vi "Flush Data to Log File.vi"(8 "error in (no error)":errorcluster, 10 "Data Queue":refnum<queue>, 11 "Logging Configuration":T1) -> (0 "error out":errorcluster)   [LabVIEW 2017, in "Logging.lvlib"]
doc: "Flush the data queue of any pending data and write it to the log file. Close the TDMS file reference."
uses:
  Logging.lvlib
  Logging Configuration.ctl
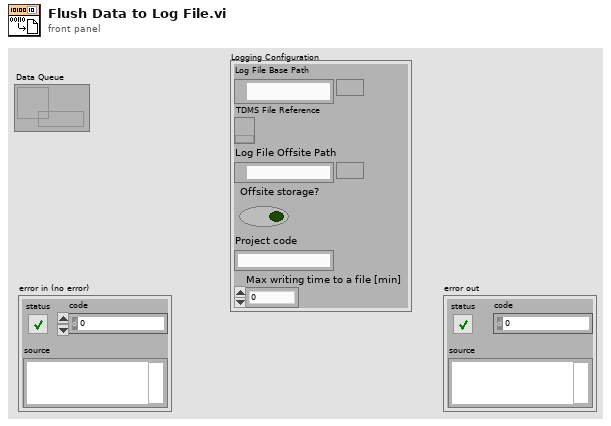
[diagram p1: front panel]
types:
  T1 = typedef "Logging.lvlib/Logging Configuration.ctl" = cluster{"Log File Base Path":path, "TDMS File Reference":refnum<k34>, "Log File Offsite Path":path, "Offsite storage?":bool, "Project code":string, "Max writing time to a file [min]":dbl}
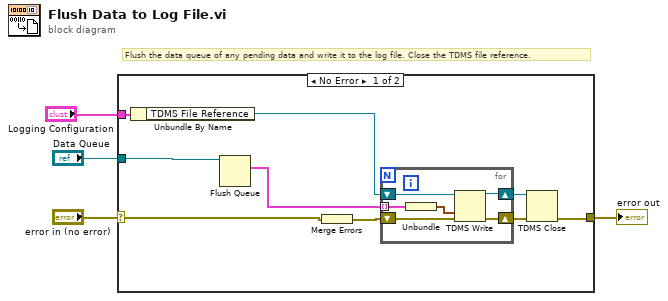
[diagram p0: block diagram]
diagram:
  # "Flush the data queue of any pending data and write it to the log file. Close the TDMS file reference."
  n1 = case shown="No Error" "error in (no error)" {
    selector: "error in (no error)" -> [w8 w20]
    tunnel: "Data Queue" -> [w10 _]
    tunnel: "Logging Configuration" -> [w6 _]
    tunnel: [w9 w20] -> w2
    frame No Error {
      n2 = Unbundle By Name(w6) -> ("TDMS File Reference"=w5:refnum<k34>)
      n3 = Flush Queue(queue=w10) -> (remaining elements=w13:cluster{"Array":waveform(dbl)[]}[])  [unwired: 1 in, 2 out]
      n4 = Merge Errors(w8) -> (w7:errorcluster)
      n5 = for {
        shift-right: [w16] -> w11
        shift-left: w5 -> [w17]
        shift-right: [w18] -> w12
        shift-left: w7 -> [w19]
        tunnel: w13 -> [w15] mode=indexing
        n6 = Unbundle(w15) -> ("Array"=w14:waveform(dbl)[])
        n7 = TDMS Write(0:w17, 9:w14, 11:w19) -> (4:w16:refnum<k34>, 15:w18:errorcluster)  [unwired: 3 in, 2 out]
      }
      n8 = TDMS Close(8:w12, 11:w11) -> (0:w9:errorcluster)  [unwired: 1 out]
    }
    frame Error {
    }
  }
  "error out" <- w2
